vi "newMain.vi"(8 "Error In":errorcluster, 9 "Zaxis Step Size":dbl, 10 "AxisID":string[](array[string]), 11 "Sim/Live":bool) -> (0 "Error Out":errorcluster, 1 "Equation":string, 2 "Three Points":dbl[][](array[numeric]), 3 "Position":dbl[](array[numeric]), 4 "D":dbl, 5 "NormalVector":dbl[](array[numeric]))   [LabVIEW 2019]
panel:
  in  "SystemID":i32
  in  "stop":bool
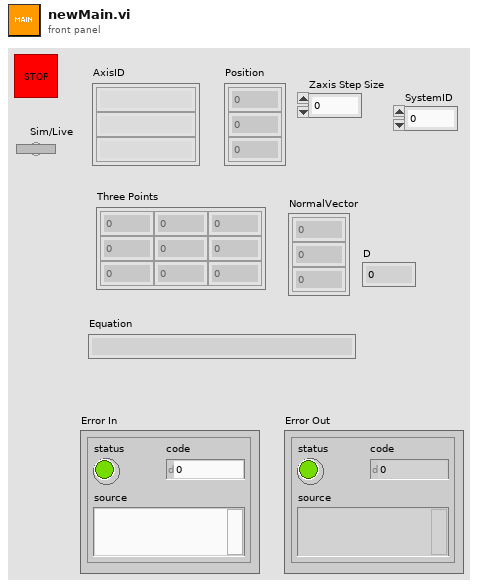
[diagram p1: front panel]
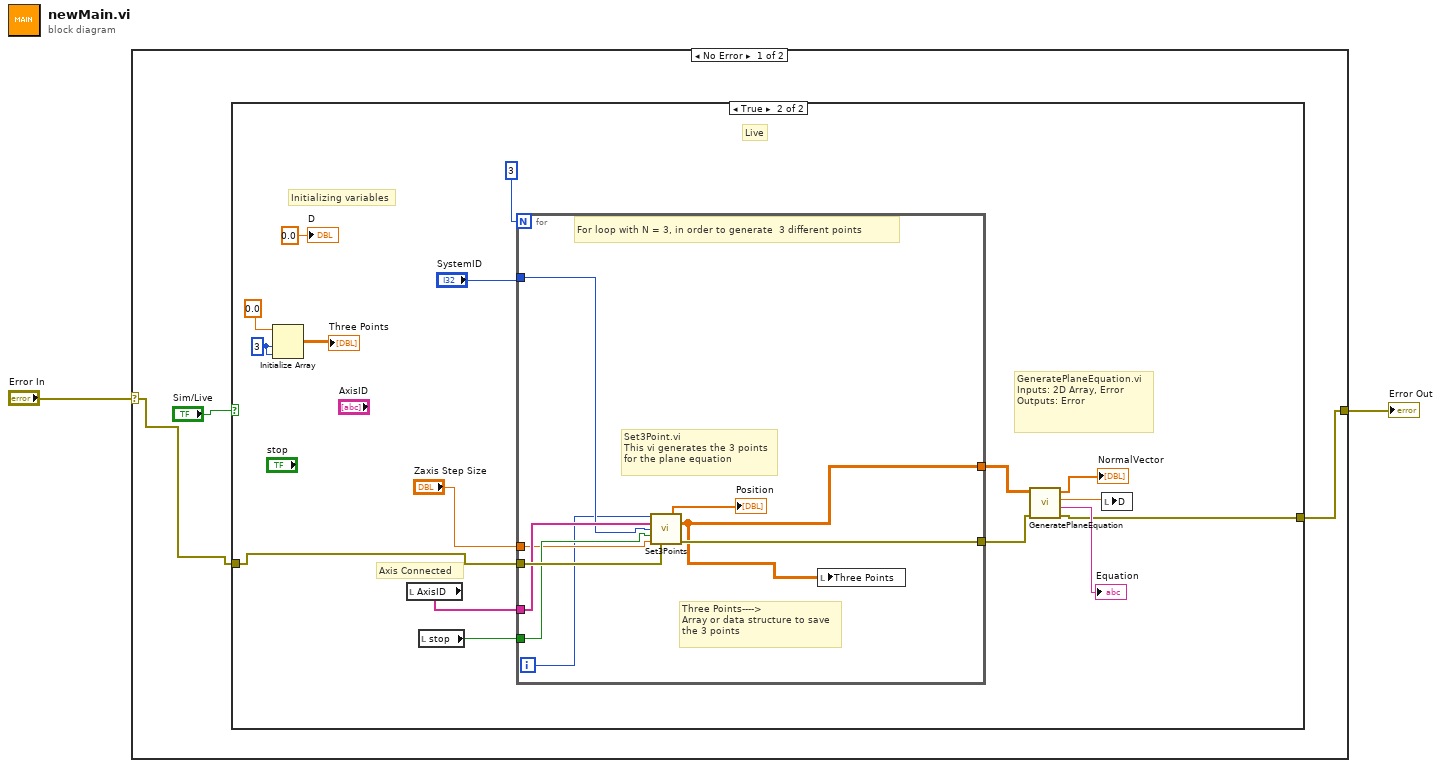
[diagram p0: block diagram]
diagram:
  n1 = case shown="No Error" "Error In" {
    selector: "Error In" -> [w4 w32]
    tunnel: [w3 w32] -> w1
    frame No Error {
      n2 = case shown="True" "Sim/Live" {
        tunnel: w4 -> [w6 w9]
        tunnel: [w6 w7] -> w3
        frame False {
          # "Simulation"
        }
        frame True {
          w12 = 3 ("dimension size")
          # "Initializing variables"
          # "Live"
          # "GeneratePlaneEquation.vi\nInputs: 2D Array, Error\nOutputs: Error"
          # "Axis Connected"
          n3 = Initialize Array(0.0 ("element"), w12, w12) -> (→"Three Points":dbl[][])
          n4 = local read "AxisID"() -> (w22:string[])
          n5 = local read "stop"() -> (w21:bool)
          n6 = for {
            N: 3 -> [_]
            tunnel: "SystemID" -> [w27]
            tunnel: w9 -> [w31]
            tunnel: w22 -> [w30]
            tunnel: w21 -> [w29]
            tunnel: "Zaxis Step Size" -> [w28]
            tunnel: [w26] -> w18
            tunnel: [w25] -> w17
            i -> [w23]
            # "Three Points---->\nArray or data structure to save\nthe 3 points"
            # "For loop with N = 3, in order to generate  3 different points"
            # "Set3Point.vi\nThis vi generates the 3 points\nfor the plane equation"
            n7 = call "Set3Points.vi"("Counter"=w23, "axis id"=w30, "System number"=w27, "stop"=w29, "Z Axis Step  Size"=w28, "Error In"=w31) -> ("Relative Position"=→"Position":dbl[], "3Points2DArray"=w25:dbl[][], "Error Out"=w26:errorcluster)  [unwired: 7 in]
            n8 = local write "Three Points"(w25) -> ()
          }
          n9 = call "GeneratePlaneEquation.vi"("Error In"=w18, "Three  points"=w17) -> ("Error Out"=w7:errorcluster, "Equation"=→"Equation":string, "D"=w15:dbl, "NormalVector"=→"NormalVector":dbl[])  [unwired: 6 in]
          n10 = local write "D"(w15) -> ()
          "D" <- 0.0 ("D")
        }
      }
    }
    frame Error {
    }
  }
  "Error Out" <- w1
